vi "ble_reset_dongle_and_cnx.vi"(8 "error in (no error)":errorcluster, 11 "COM Bluegiga in":refnum<visa-resource-name>) -> (0 "error out":errorcluster, 3 "COM Bluegiga out":refnum<visa-resource-name>)   [LabVIEW 2017]
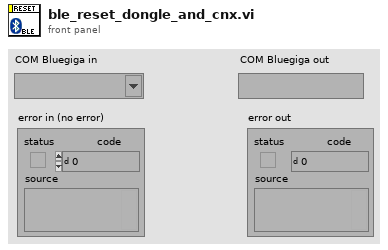
[diagram p1: front panel]
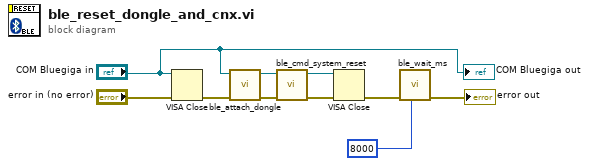
[diagram p0: block diagram]
diagram:
  n1 = VISA Close(VISA resource name="COM Bluegiga in", error in (no error)="error in (no error)") -> (error out=w4:errorcluster)
  n2 = call "ble_attach_dongle.vi"("error in (no error)"=w4, "COM Bluegiga in"="COM Bluegiga in") -> ("error out"=w5:errorcluster, "COM Bluegiga out"=w6:refnum<visa-resource-name>)  [unwired: 8 in]
  n3 = call "ble_cmd_system_reset.vi"("error in (no error)"=w5, "COM Bluegiga in"=w6) -> ("error out"=w8:errorcluster, "COM Bluegiga out"=w9:refnum<visa-resource-name>)  [unwired: 8 in]
  n4 = VISA Close(VISA resource name=w9, error in (no error)=w8) -> (error out=w10:errorcluster)
  n5 = call "ble_wait_ms.vi"("milliseconds to wait (100)"=u32 8000, "error in (no error)"=w10) -> ("error out"=→"error out":errorcluster)  [unwired: 9 in]
  "COM Bluegiga out" <- "COM Bluegiga in"
